vi "Prueba Trip Gap.vi"(11 "Class 2.lvclass":refnum<class "Class 2.lvclass">) -> (3 "Class 2.lvclass 2":refnum<class "Class 2.lvclass">)   [LabVIEW 2019, in "Class 2.lvclass"]
uses:
  Class 2.lvclass
  Class 2.lvclass/Class 2.ctl
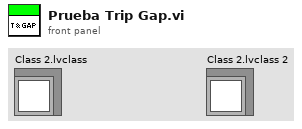
[diagram p1: front panel]
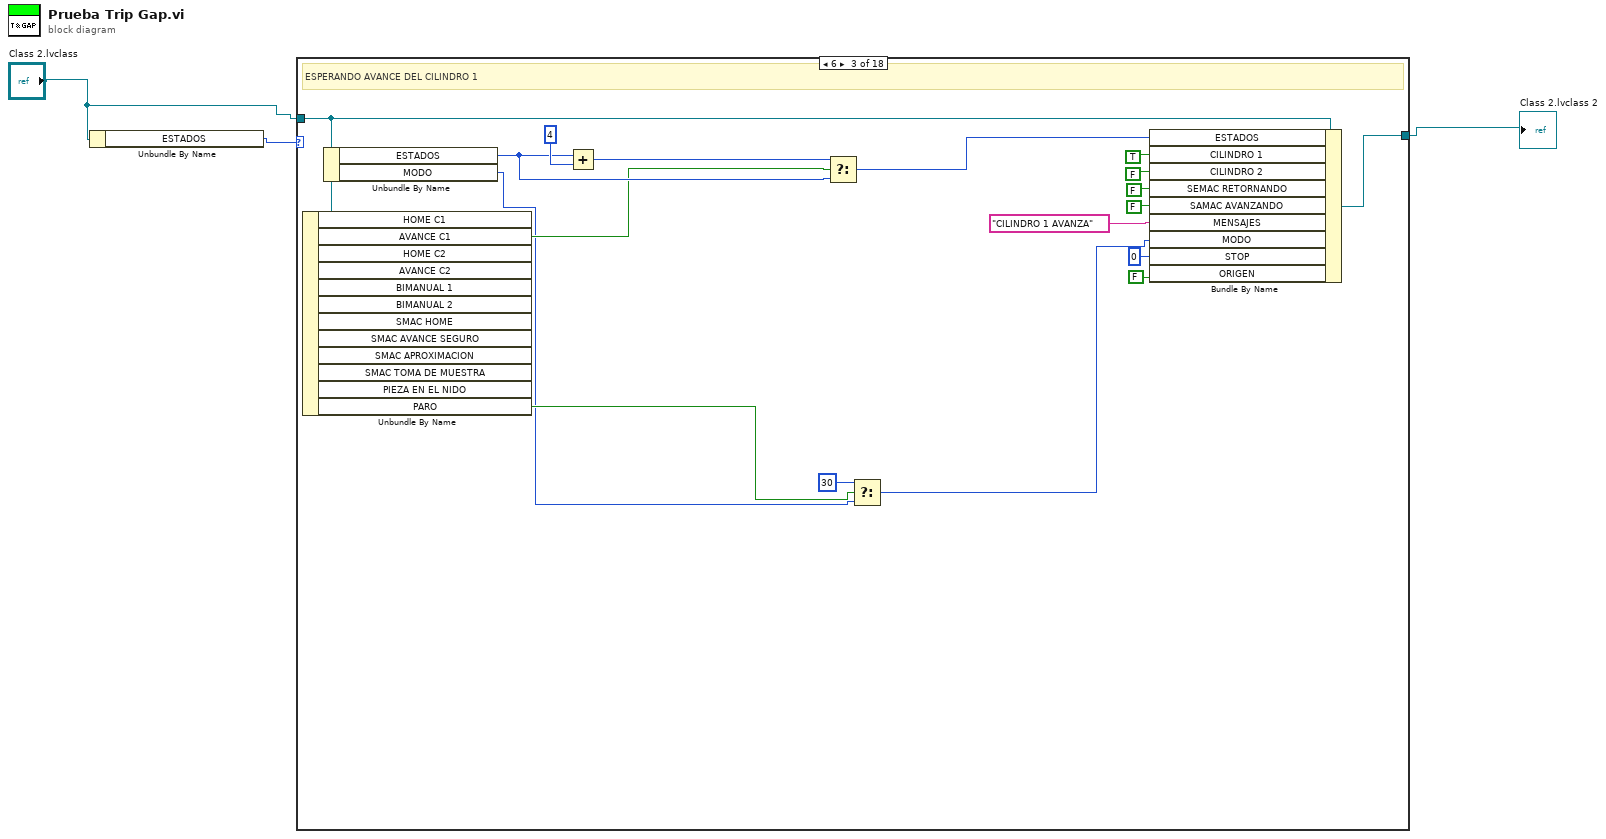
[diagram p0: block diagram]
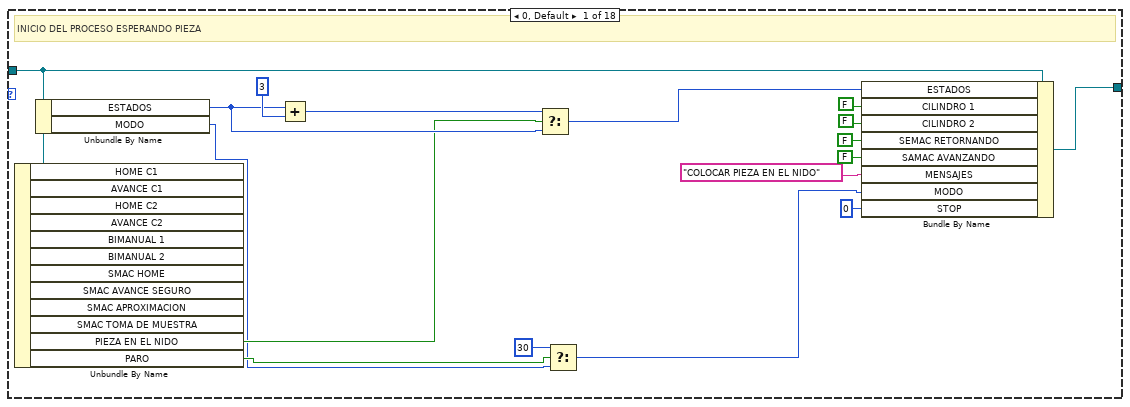
[diagram p2: hidden frame]
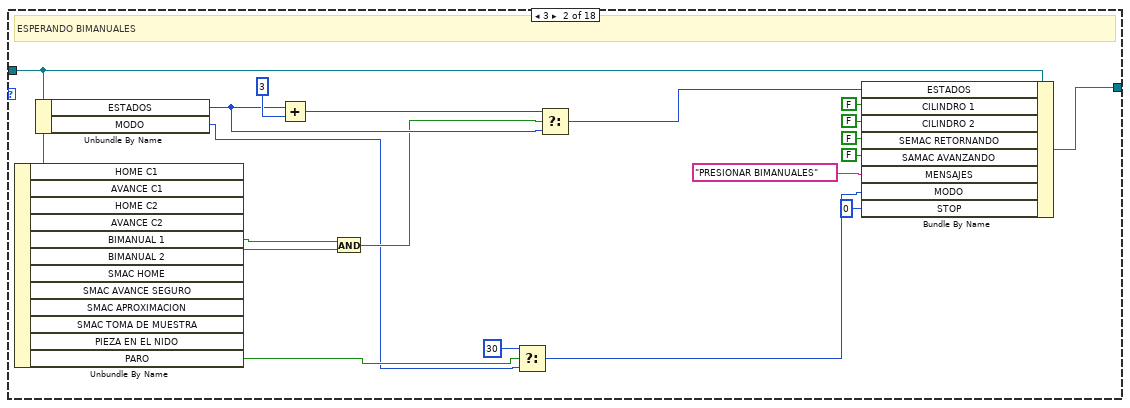
[diagram p3: hidden frame]
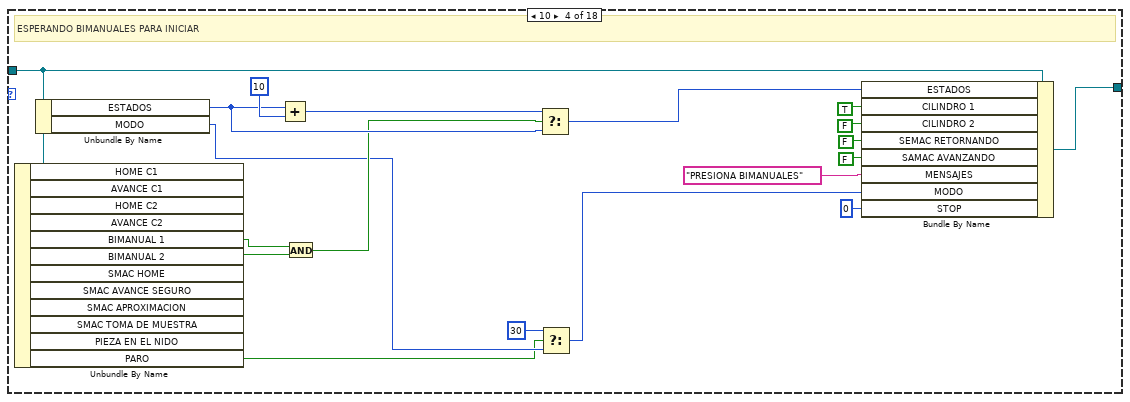
[diagram p4: hidden frame]
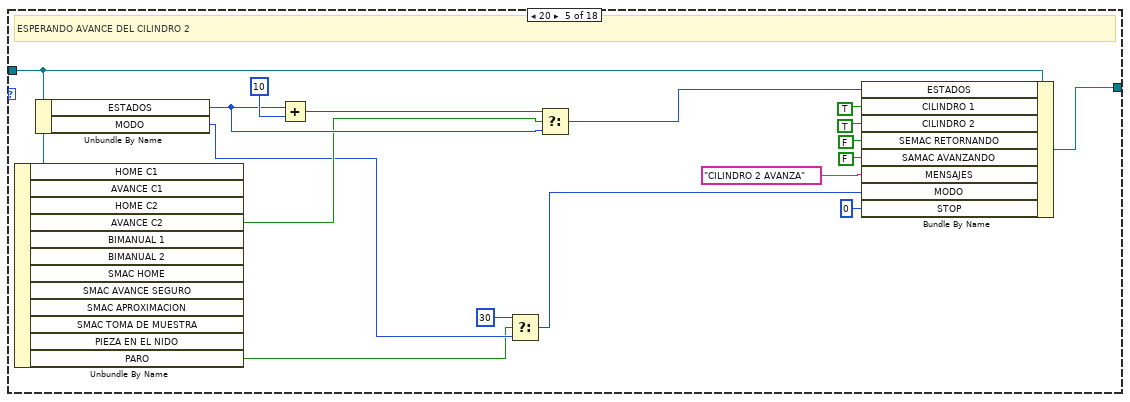
[diagram p5: hidden frame]
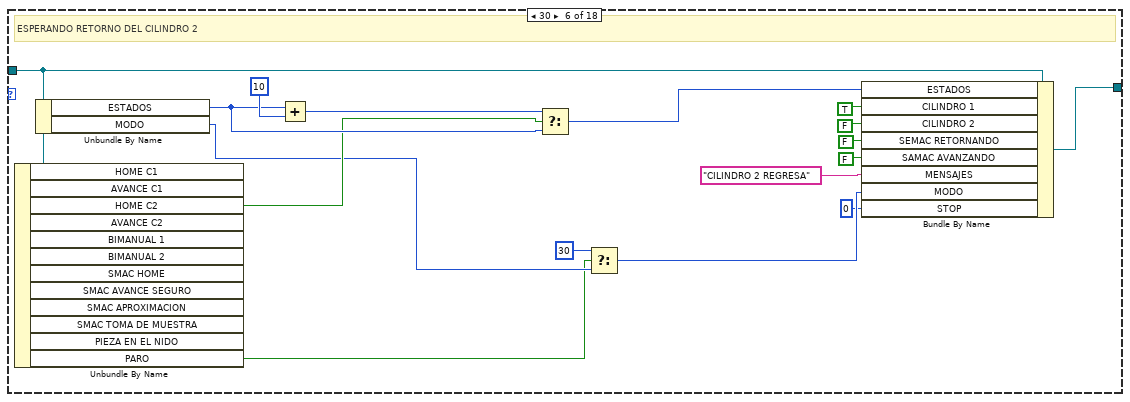
[diagram p6: hidden frame]
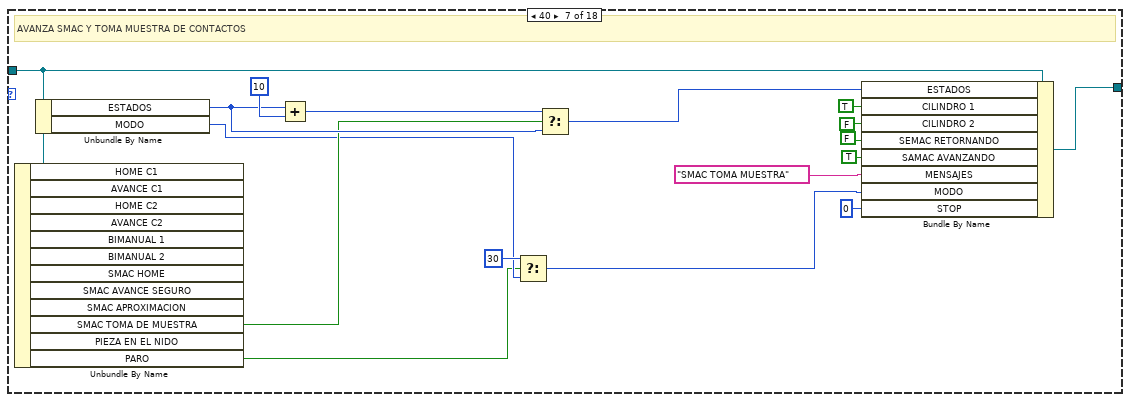
[diagram p7: hidden frame]
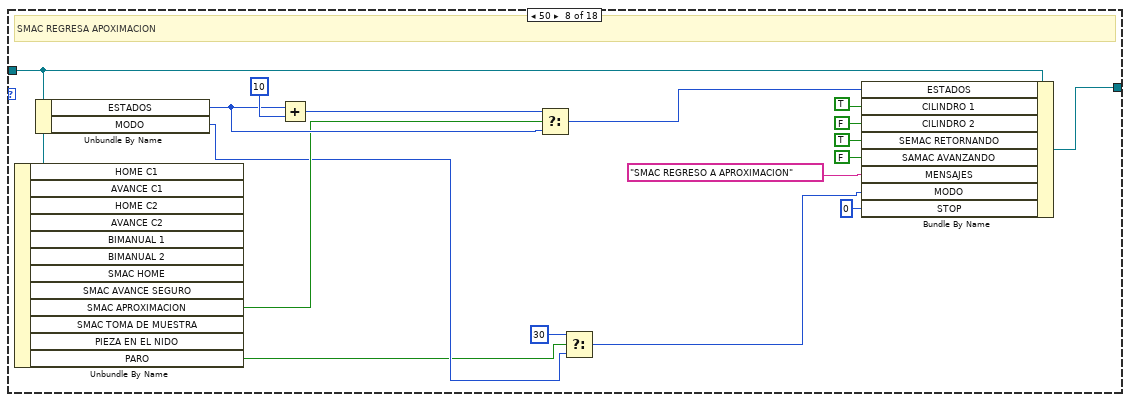
[diagram p8: hidden frame]
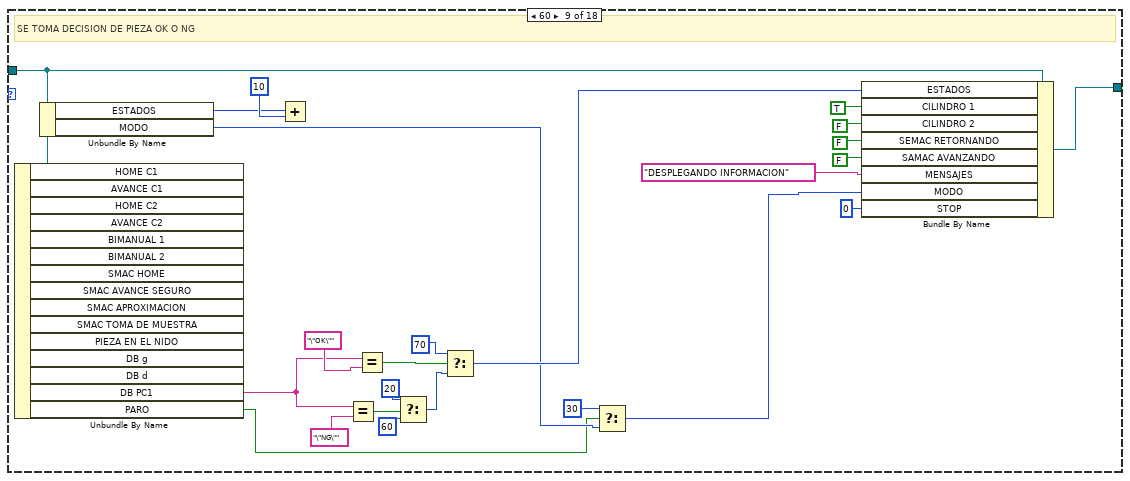
[diagram p9: hidden frame]
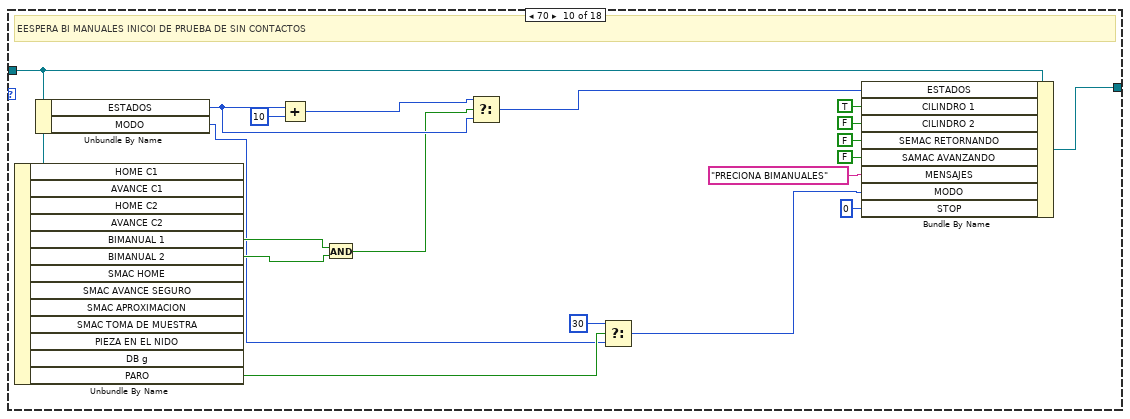
[diagram p10: hidden frame]
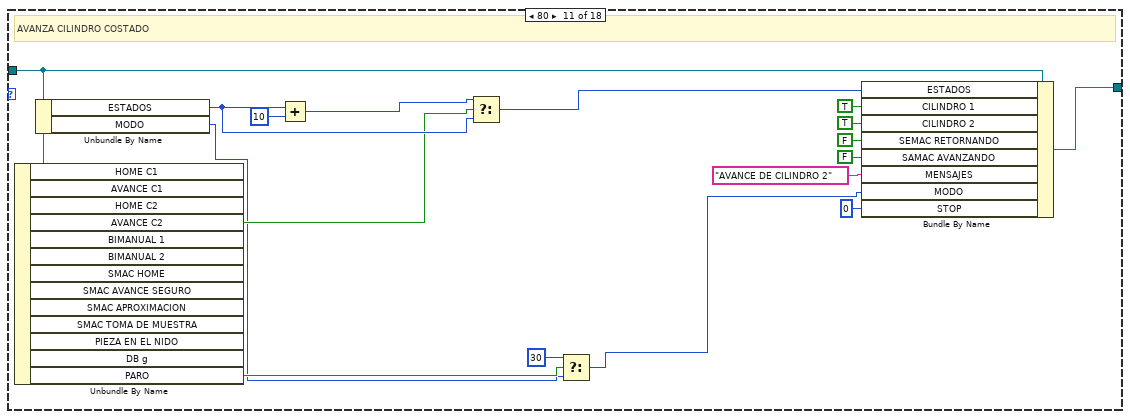
[diagram p11: hidden frame]
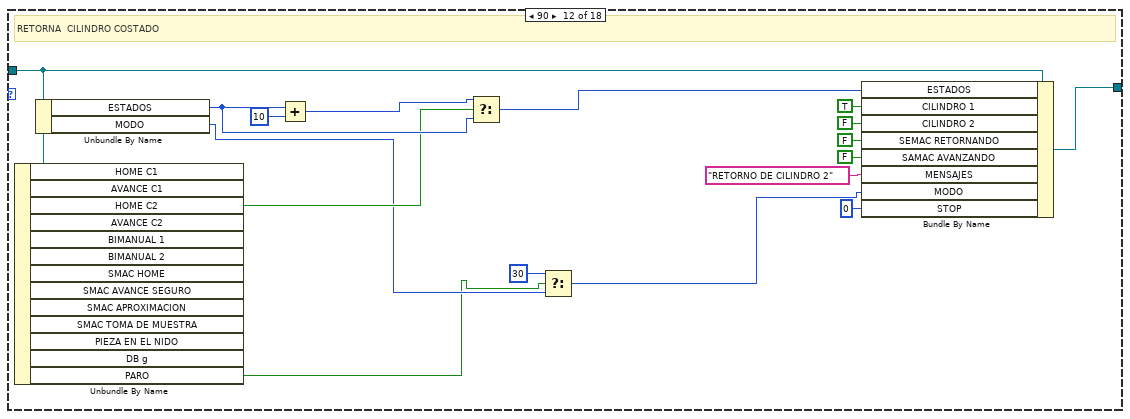
[diagram p12: hidden frame]
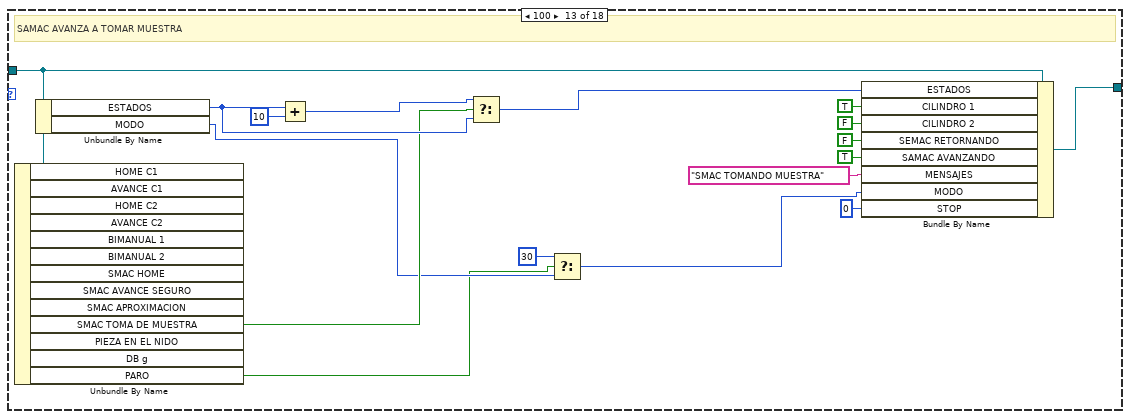
[diagram p13: hidden frame]
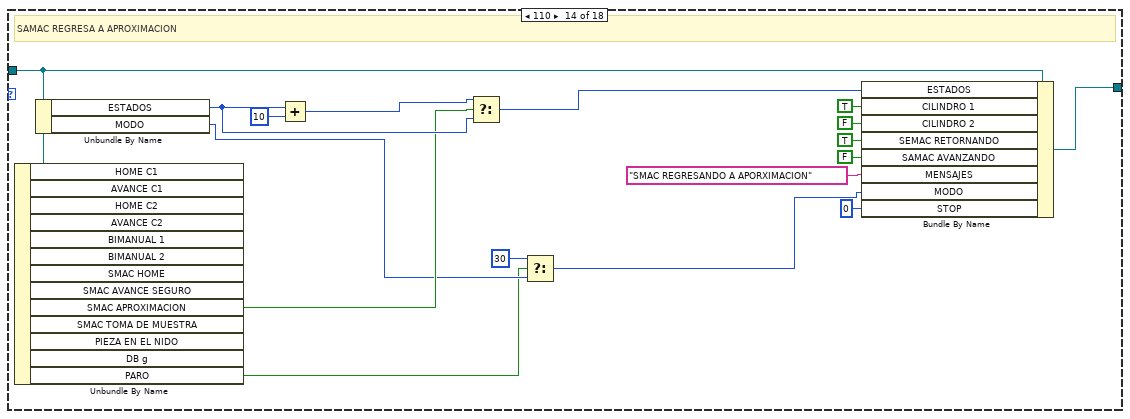
[diagram p14: hidden frame]
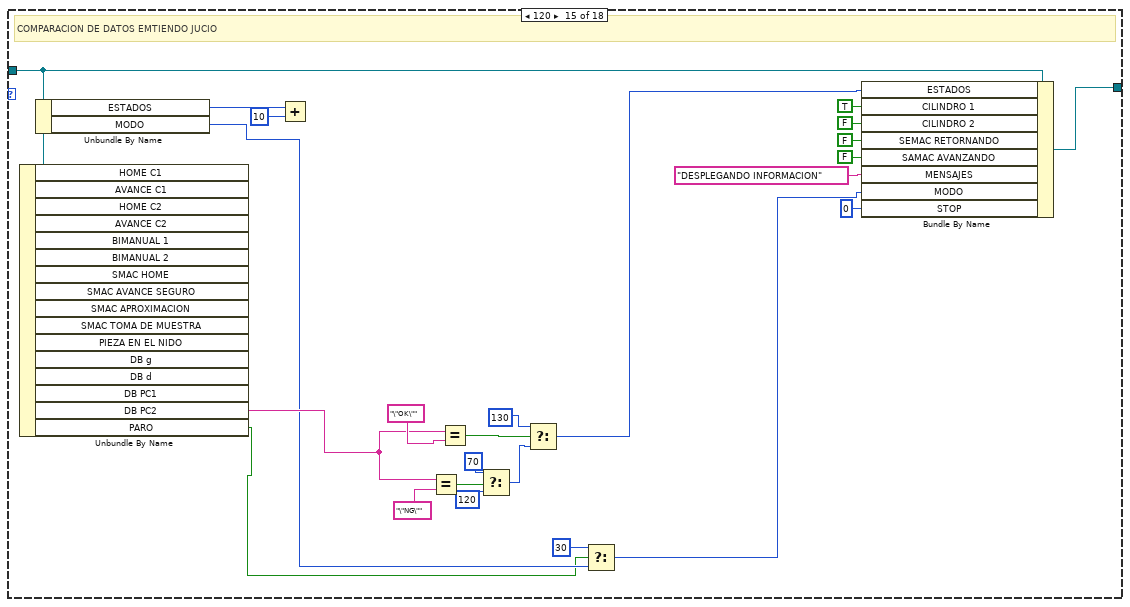
[diagram p15: hidden frame]
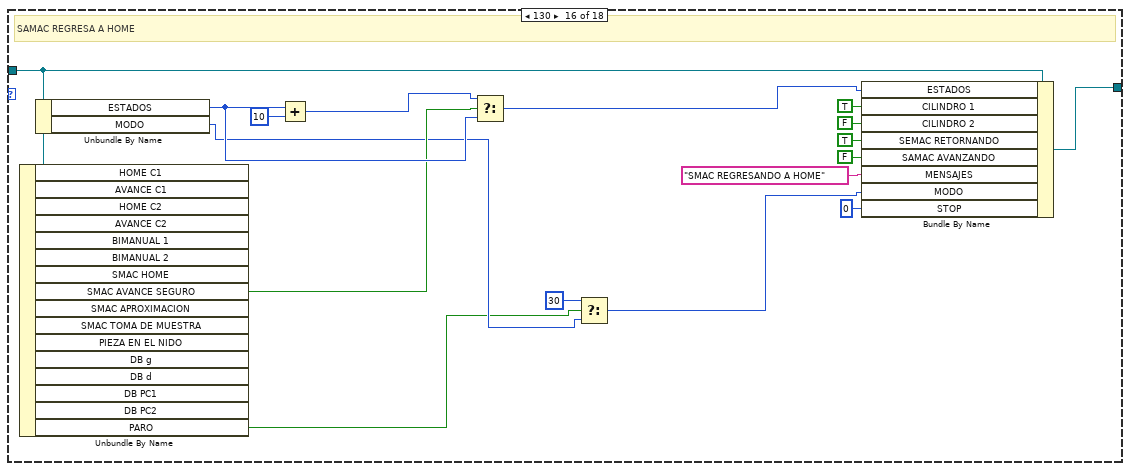
[diagram p16: hidden frame]
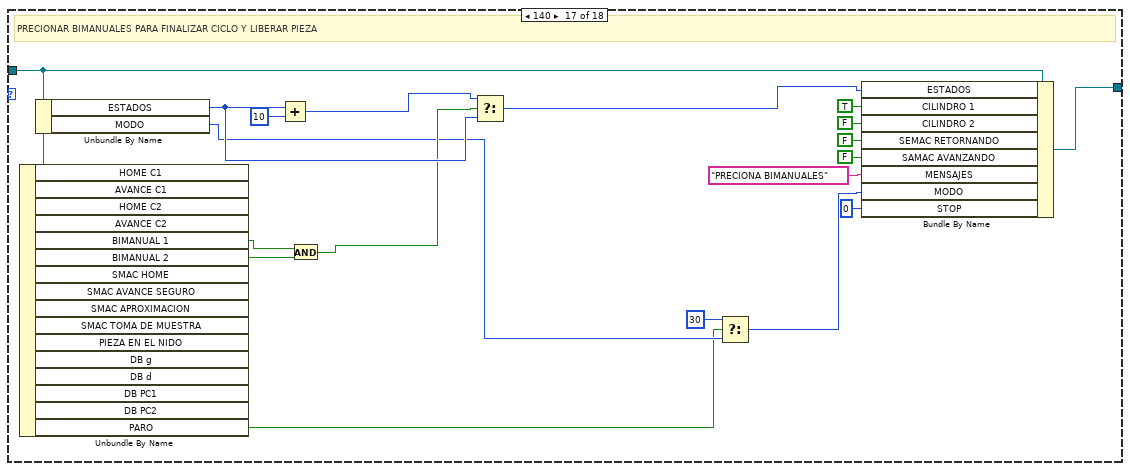
[diagram p17: hidden frame]
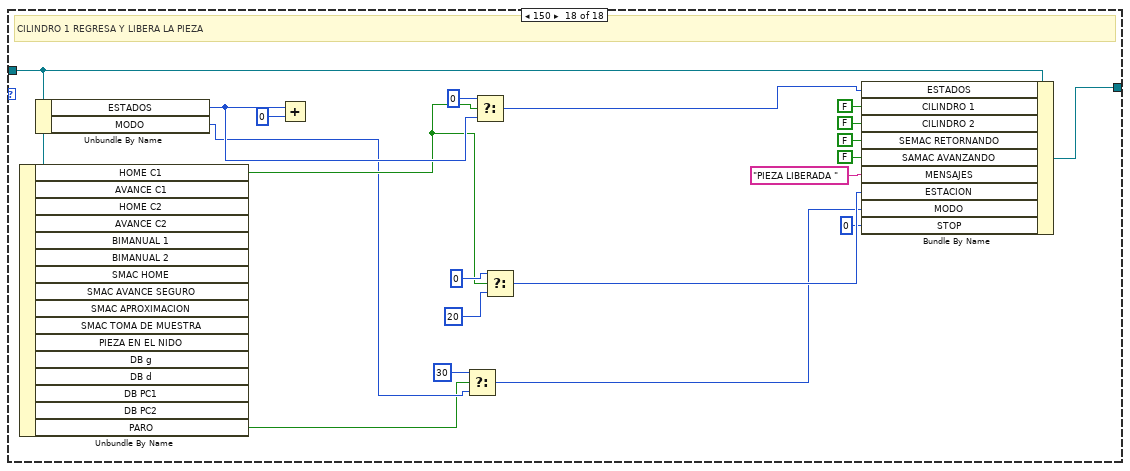
[diagram p18: hidden frame]
diagram:
  n1 = Unbundle By Name("Class 2.lvclass") -> ("ESTADOS"=w3:i16)
  n2 = case shown="6" w3 {
    tunnel: "Class 2.lvclass" -> [w15 w34 w52 w71 w88 w105 w122 w139 w166 w185 w202 w219 w236 w253 w277 w294 w313 w333]
    tunnel: [w20 w39 w57 w76 w93 w110 w127 w144 w168 w187 w204 w221 w238 w255 w279 w296 w315 w335] -> w1
    frame 0, Default {
      # "INICIO DEL PROCESO ESPERANDO PIEZA"
      n3 = Unbundle By Name(w15) -> ("PIEZA EN EL NIDO"=w13:bool, "PARO"=w5:bool)  [unwired: 10 out]
      n4 = Unbundle By Name(w15) -> ("ESTADOS"=w17:i16, "MODO"=w4:i16)
      n5 = Add(x=w17, y=i16 3) -> (x+y=w18:i16)
      n6 = Select(t=w18, s=w13, f=w17) -> (s? t:f=w16:i16)
      n7 = Select(t=i16 30, s=w5, f=w4) -> (s? t:f=w7:i16)
      n8 = Bundle By Name(cluster=w15, "ESTADOS"=w16, "CILINDRO 1"=FALSE ("SALIDAS.CILINDRO 1"), "CILINDRO 2"=FALSE ("SALIDAS.CILINDRO 2"), "SEMAC RETORNANDO"=FALSE ("SALIDAS.SEMAC RETORNANDO"), "SAMAC AVANZANDO"=FALSE ("SALIDAS.SAMAC AVANZANDO"), "MENSAJES"="COLOCAR PIEZA EN EL NIDO" ("SALIDAS.MENSAJES"), "MODO"=w7, "STOP"=i16 0 ("MAQ DE ESTADOS.STOP")) -> (w20:refnum<class "Class 2.lvclass">)
    }
    frame 3 {
      # "ESPERANDO BIMANUALES"
      n9 = Unbundle By Name(w34) -> ("BIMANUAL 1"=w28:bool, "BIMANUAL 2"=w27:bool, "PARO"=w22:bool)  [unwired: 9 out]
      n10 = Unbundle By Name(w34) -> ("ESTADOS"=w36:i16, "MODO"=w21:i16)
      n11 = Add(x=w36, y=i16 3) -> (x+y=w37:i16)
      n12 = And(x=w28, y=w27) -> (x .and. y?=w26:bool)
      n13 = Select(t=i16 30, s=w22, f=w21) -> (s? t:f=w24:i16)
      n14 = Select(t=w37, s=w26, f=w36) -> (s? t:f=w35:i16)
      n15 = Bundle By Name(cluster=w34, "ESTADOS"=w35, "CILINDRO 1"=FALSE ("SALIDAS.CILINDRO 1"), "CILINDRO 2"=FALSE ("SALIDAS.CILINDRO 2"), "SEMAC RETORNANDO"=FALSE ("SALIDAS.SEMAC RETORNANDO"), "SAMAC AVANZANDO"=FALSE ("SALIDAS.SAMAC AVANZANDO"), "MENSAJES"="PRESIONAR BIMANUALES" ("SALIDAS.MENSAJES"), "MODO"=w24, "STOP"=i16 0 ("MAQ DE ESTADOS.STOP")) -> (w39:refnum<class "Class 2.lvclass">)
    }
    frame 6 {
      # "ESPERANDO AVANCE DEL CILINDRO 1"
      n16 = Unbundle By Name(w52) -> ("AVANCE C1"=w46:bool, "PARO"=w42:bool)  [unwired: 10 out]
      n17 = Unbundle By Name(w52) -> ("ESTADOS"=w54:i16, "MODO"=w41:i16)
      n18 = Add(x=w54, y=i16 4) -> (x+y=w55:i16)
      n19 = Select(t=w55, s=w46, f=w54) -> (s? t:f=w53:i16)
      n20 = Select(t=i16 30, s=w42, f=w41) -> (s? t:f=w44:i16)
      n21 = Bundle By Name(cluster=w52, "ESTADOS"=w53, "CILINDRO 1"=TRUE ("SALIDAS.CILINDRO 1"), "CILINDRO 2"=FALSE ("SALIDAS.CILINDRO 2"), "SEMAC RETORNANDO"=FALSE ("SALIDAS.SEMAC RETORNANDO"), "SAMAC AVANZANDO"=FALSE ("SALIDAS.SAMAC AVANZANDO"), "MENSAJES"="CILINDRO 1 AVANZA" ("SALIDAS.MENSAJES"), "MODO"=w44, "STOP"=i16 0 ("MAQ DE ESTADOS.STOP"), "ORIGEN"=FALSE ("PROCESO.ORIGEN")) -> (w57:refnum<class "Class 2.lvclass">)
    }
    frame 10 {
      # "ESPERANDO BIMANUALES PARA INICIAR"
      n22 = Unbundle By Name(w71) -> ("BIMANUAL 1"=w65:bool, "BIMANUAL 2"=w64:bool, "PARO"=w58:bool)  [unwired: 9 out]
      n23 = Unbundle By Name(w71) -> ("ESTADOS"=w73:i16, "MODO"=w59:i16)
      n24 = Add(x=w73, y=i16 10) -> (x+y=w74:i16)
      n25 = And(x=w65, y=w64) -> (x .and. y?=w63:bool)
      n26 = Select(t=w74, s=w63, f=w73) -> (s? t:f=w72:i16)
      n27 = Select(t=i16 30, s=w58, f=w59) -> (s? t:f=w61:i16)
      n28 = Bundle By Name(cluster=w71, "ESTADOS"=w72, "CILINDRO 1"=TRUE ("SALIDAS.CILINDRO 1"), "CILINDRO 2"=FALSE ("SALIDAS.CILINDRO 2"), "SEMAC RETORNANDO"=FALSE ("SALIDAS.SEMAC RETORNANDO"), "SAMAC AVANZANDO"=FALSE ("SALIDAS.SAMAC AVANZANDO"), "MENSAJES"="PRESIONA BIMANUALES" ("SALIDAS.MENSAJES"), "MODO"=w61, "STOP"=i16 0 ("MAQ DE ESTADOS.STOP")) -> (w76:refnum<class "Class 2.lvclass">)
    }
    frame 20 {
      # "ESPERANDO AVANCE DEL CILINDRO 2"
      n29 = Unbundle By Name(w88) -> ("AVANCE C2"=w82:bool, "PARO"=w77:bool)  [unwired: 10 out]
      n30 = Unbundle By Name(w88) -> ("ESTADOS"=w90:i16, "MODO"=w78:i16)
      n31 = Add(x=w90, y=i16 10) -> (x+y=w91:i16)
      n32 = Select(t=i16 30, s=w77, f=w78) -> (s? t:f=w80:i16)
      n33 = Select(t=w91, s=w82, f=w90) -> (s? t:f=w89:i16)
      n34 = Bundle By Name(cluster=w88, "ESTADOS"=w89, "CILINDRO 1"=TRUE ("SALIDAS.CILINDRO 1"), "CILINDRO 2"=TRUE ("SALIDAS.CILINDRO 2"), "SEMAC RETORNANDO"=FALSE ("SALIDAS.SEMAC RETORNANDO"), "SAMAC AVANZANDO"=FALSE ("SALIDAS.SAMAC AVANZANDO"), "MENSAJES"="CILINDRO 2 AVANZA" ("SALIDAS.MENSAJES"), "MODO"=w80, "STOP"=i16 0 ("MAQ DE ESTADOS.STOP")) -> (w93:refnum<class "Class 2.lvclass">)
    }
    frame 30 {
      # "ESPERANDO RETORNO DEL CILINDRO 2"
      n35 = Unbundle By Name(w105) -> ("HOME C2"=w99:bool, "PARO"=w94:bool)  [unwired: 10 out]
      n36 = Unbundle By Name(w105) -> ("ESTADOS"=w107:i16, "MODO"=w95:i16)
      n37 = Add(x=w107, y=i16 10) -> (x+y=w108:i16)
      n38 = Select(t=w108, s=w99, f=w107) -> (s? t:f=w106:i16)
      n39 = Select(t=i16 30, s=w94, f=w95) -> (s? t:f=w97:i16)
      n40 = Bundle By Name(cluster=w105, "ESTADOS"=w106, "CILINDRO 1"=TRUE ("SALIDAS.CILINDRO 1"), "CILINDRO 2"=FALSE ("SALIDAS.CILINDRO 2"), "SEMAC RETORNANDO"=FALSE ("SALIDAS.SEMAC RETORNANDO"), "SAMAC AVANZANDO"=FALSE ("SALIDAS.SAMAC AVANZANDO"), "MENSAJES"="CILINDRO 2 REGRESA" ("SALIDAS.MENSAJES"), "MODO"=w97, "STOP"=i16 0 ("MAQ DE ESTADOS.STOP")) -> (w110:refnum<class "Class 2.lvclass">)
    }
    frame 40 {
      # "AVANZA SMAC Y TOMA MUESTRA DE CONTACTOS"
      n41 = Unbundle By Name(w122) -> ("SMAC TOMA DE MUESTRA"=w116:bool, "PARO"=w111:bool)  [unwired: 10 out]
      n42 = Unbundle By Name(w122) -> ("ESTADOS"=w124:i16, "MODO"=w112:i16)
      n43 = Add(x=w124, y=i16 10) -> (x+y=w125:i16)
      n44 = Select(t=i16 30, s=w111, f=w112) -> (s? t:f=w114:i16)
      n45 = Select(t=w125, s=w116, f=w124) -> (s? t:f=w123:i16)
      n46 = Bundle By Name(cluster=w122, "ESTADOS"=w123, "CILINDRO 1"=TRUE ("SALIDAS.CILINDRO 1"), "CILINDRO 2"=FALSE ("SALIDAS.CILINDRO 2"), "SEMAC RETORNANDO"=FALSE ("SALIDAS.SEMAC RETORNANDO"), "SAMAC AVANZANDO"=TRUE ("SALIDAS.SAMAC AVANZANDO"), "MENSAJES"="SMAC TOMA MUESTRA" ("SALIDAS.MENSAJES"), "MODO"=w114, "STOP"=i16 0 ("MAQ DE ESTADOS.STOP")) -> (w127:refnum<class "Class 2.lvclass">)
    }
    frame 50 {
      # "SMAC REGRESA APOXIMACION"
      n47 = Unbundle By Name(w139) -> ("SMAC APROXIMACION"=w133:bool, "PARO"=w128:bool)  [unwired: 10 out]
      n48 = Unbundle By Name(w139) -> ("ESTADOS"=w141:i16, "MODO"=w129:i16)
      n49 = Add(x=w141, y=i16 10) -> (x+y=w142:i16)
      n50 = Select(t=w142, s=w133, f=w141) -> (s? t:f=w140:i16)
      n51 = Select(t=i16 30, s=w128, f=w129) -> (s? t:f=w131:i16)
      n52 = Bundle By Name(cluster=w139, "ESTADOS"=w140, "CILINDRO 1"=TRUE ("SALIDAS.CILINDRO 1"), "CILINDRO 2"=FALSE ("SALIDAS.CILINDRO 2"), "SEMAC RETORNANDO"=TRUE ("SALIDAS.SEMAC RETORNANDO"), "SAMAC AVANZANDO"=FALSE ("SALIDAS.SAMAC AVANZANDO"), "MENSAJES"="SMAC REGRESO A APROXIMACION" ("SALIDAS.MENSAJES"), "MODO"=w131, "STOP"=i16 0 ("MAQ DE ESTADOS.STOP")) -> (w144:refnum<class "Class 2.lvclass">)
    }
    frame 60 {
      # "SE TOMA DECISION DE PIEZA OK O NG"
      n53 = Unbundle By Name(w166) -> ("DB PC1"=w150:string, "PARO"=w145:bool)  [unwired: 13 out]
      n54 = Unbundle By Name(w166) -> ("ESTADOS"=w159:i16, "MODO"=w146:i16)
      n55 = Add(x=w159, y=i16 10) -> ()  [unwired: 1 out]
      n56 = Equal?(x=w150, y="\"NG\"") -> (x = y?=w157:bool)
      n57 = Equal?(x=w150, y="\"OK\"") -> (x = y?=w158:bool)
      n58 = Select(t=i16 20 ("y"), s=w157, f=i16 60) -> (s? t:f=w154:i16)
      n59 = Select(t=i16 70, s=w158, f=w154) -> (s? t:f=w152:i16)
      n60 = Select(t=i16 30, s=w145, f=w146) -> (s? t:f=w148:i16)
      n61 = Bundle By Name(cluster=w166, "ESTADOS"=w152, "CILINDRO 1"=TRUE ("SALIDAS.CILINDRO 1"), "CILINDRO 2"=FALSE ("SALIDAS.CILINDRO 2"), "SEMAC RETORNANDO"=FALSE ("SALIDAS.SEMAC RETORNANDO"), "SAMAC AVANZANDO"=FALSE ("SALIDAS.SAMAC AVANZANDO"), "MENSAJES"="DESPLEGANDO INFORMACION" ("SALIDAS.MENSAJES"), "MODO"=w148, "STOP"=i16 0 ("MAQ DE ESTADOS.MODO")) -> (w168:refnum<class "Class 2.lvclass">)
    }
    frame 70 {
      # "EESPERA BI MANUALES INICOI DE PRUEBA DE SIN CONTACTOS"
      n62 = Unbundle By Name(w185) -> ("BIMANUAL 1"=w176:bool, "BIMANUAL 2"=w175:bool, "PARO"=w172:bool)  [unwired: 10 out]
      n63 = Unbundle By Name(w185) -> ("ESTADOS"=w178:i16, "MODO"=w171:i16)
      n64 = Add(x=w178, y=i16 10) -> (x+y=w177:i16)
      n65 = And(x=w176, y=w175) -> (x .and. y?=w174:bool)
      n66 = Select(t=w177, s=w174, f=w178) -> (s? t:f=w179:i16)
      n67 = Select(t=i16 30, s=w172, f=w171) -> (s? t:f=w170:i16)
      n68 = Bundle By Name(cluster=w185, "ESTADOS"=w179, "CILINDRO 1"=TRUE ("SALIDAS.CILINDRO 1"), "CILINDRO 2"=FALSE ("SALIDAS.CILINDRO 2"), "SEMAC RETORNANDO"=FALSE ("SALIDAS.SEMAC RETORNANDO"), "SAMAC AVANZANDO"=FALSE ("SALIDAS.SAMAC AVANZANDO"), "MENSAJES"="PRECIONA BIMANUALES" ("SALIDAS.MENSAJES"), "MODO"=w170, "STOP"=i16 0 ("MAQ DE ESTADOS.STOP")) -> (w187:refnum<class "Class 2.lvclass">)
    }
    frame 80 {
      # "AVANZA CILINDRO COSTADO"
      n69 = Unbundle By Name(w202) -> ("AVANCE C2"=w193:bool, "PARO"=w191:bool)  [unwired: 11 out]
      n70 = Unbundle By Name(w202) -> ("ESTADOS"=w195:i16, "MODO"=w190:i16)
      n71 = Add(x=w195, y=i16 10) -> (x+y=w194:i16)
      n72 = Select(t=w194, s=w193, f=w195) -> (s? t:f=w196:i16)
      n73 = Select(t=i16 30, s=w191, f=w190) -> (s? t:f=w189:i16)
      n74 = Bundle By Name(cluster=w202, "ESTADOS"=w196, "CILINDRO 1"=TRUE ("SALIDAS.CILINDRO 1"), "CILINDRO 2"=TRUE ("SALIDAS.CILINDRO 2"), "SEMAC RETORNANDO"=FALSE ("SALIDAS.SEMAC RETORNANDO"), "SAMAC AVANZANDO"=FALSE ("SALIDAS.SAMAC AVANZANDO"), "MENSAJES"="AVANCE DE CILINDRO 2" ("SALIDAS.MENSAJES"), "MODO"=w189, "STOP"=i16 0 ("MAQ DE ESTADOS.STOP")) -> (w204:refnum<class "Class 2.lvclass">)
    }
    frame 90 {
      # "RETORNA  CILINDRO COSTADO"
      n75 = Unbundle By Name(w219) -> ("HOME C2"=w210:bool, "PARO"=w206:bool)  [unwired: 11 out]
      n76 = Unbundle By Name(w219) -> ("ESTADOS"=w212:i16, "MODO"=w207:i16)
      n77 = Add(x=w212, y=i16 10) -> (x+y=w211:i16)
      n78 = Select(t=w211, s=w210, f=w212) -> (s? t:f=w213:i16)
      n79 = Select(t=i16 30, s=w206, f=w207) -> (s? t:f=w208:i16)
      n80 = Bundle By Name(cluster=w219, "ESTADOS"=w213, "CILINDRO 1"=TRUE ("SALIDAS.CILINDRO 1"), "CILINDRO 2"=FALSE ("SALIDAS.CILINDRO 2"), "SEMAC RETORNANDO"=FALSE ("SALIDAS.SEMAC RETORNANDO"), "SAMAC AVANZANDO"=FALSE ("SALIDAS.SAMAC AVANZANDO"), "MENSAJES"="RETORNO DE CILINDRO 2" ("SALIDAS.MENSAJES"), "MODO"=w208, "STOP"=i16 0 ("MAQ DE ESTADOS.STOP")) -> (w221:refnum<class "Class 2.lvclass">)
    }
    frame 100 {
      # "SAMAC AVANZA A TOMAR MUESTRA"
      n81 = Unbundle By Name(w236) -> ("SMAC TOMA DE MUESTRA"=w227:bool, "PARO"=w222:bool)  [unwired: 11 out]
      n82 = Unbundle By Name(w236) -> ("ESTADOS"=w229:i16, "MODO"=w223:i16)
      n83 = Add(x=w229, y=i16 10) -> (x+y=w228:i16)
      n84 = Select(t=w228, s=w227, f=w229) -> (s? t:f=w230:i16)
      n85 = Select(t=i16 30, s=w222, f=w223) -> (s? t:f=w225:i16)
      n86 = Bundle By Name(cluster=w236, "ESTADOS"=w230, "CILINDRO 1"=TRUE ("SALIDAS.CILINDRO 1"), "CILINDRO 2"=FALSE ("SALIDAS.CILINDRO 2"), "SEMAC RETORNANDO"=FALSE ("SALIDAS.SEMAC RETORNANDO"), "SAMAC AVANZANDO"=TRUE ("SALIDAS.SAMAC AVANZANDO"), "MENSAJES"="SMAC TOMANDO MUESTRA" ("SALIDAS.MENSAJES"), "MODO"=w225, "STOP"=i16 0 ("MAQ DE ESTADOS.STOP")) -> (w238:refnum<class "Class 2.lvclass">)
    }
    frame 110 {
      # "SAMAC REGRESA A APROXIMACION"
      n87 = Unbundle By Name(w253) -> ("SMAC APROXIMACION"=w244:bool, "PARO"=w239:bool)  [unwired: 11 out]
      n88 = Unbundle By Name(w253) -> ("ESTADOS"=w246:i16, "MODO"=w240:i16)
      n89 = Add(x=w246, y=i16 10) -> (x+y=w245:i16)
      n90 = Select(t=w245, s=w244, f=w246) -> (s? t:f=w247:i16)
      n91 = Select(t=i16 30, s=w239, f=w240) -> (s? t:f=w242:i16)
      n92 = Bundle By Name(cluster=w253, "ESTADOS"=w247, "CILINDRO 1"=TRUE ("SALIDAS.CILINDRO 1"), "CILINDRO 2"=FALSE ("SALIDAS.CILINDRO 2"), "SEMAC RETORNANDO"=TRUE ("SALIDAS.SEMAC RETORNANDO"), "SAMAC AVANZANDO"=FALSE ("SALIDAS.SAMAC AVANZANDO"), "MENSAJES"="SMAC REGRESANDO A APORXIMACION" ("SALIDAS.MENSAJES"), "MODO"=w242, "STOP"=i16 0 ("MAQ DE ESTADOS.STOP")) -> (w255:refnum<class "Class 2.lvclass">)
    }
    frame 120 {
      # "COMPARACION DE DATOS EMTIENDO JUCIO"
      n93 = Unbundle By Name(w277) -> ("DB PC2"=w262:string, "PARO"=w256:bool)  [unwired: 14 out]
      n94 = Unbundle By Name(w277) -> ("ESTADOS"=w271:i16, "MODO"=w257:i16)
      n95 = Add(x=w271, y=i16 10) -> ()  [unwired: 1 out]
      n96 = Equal?(x=w262, y="\"NG\"") -> (x = y?=w268:bool)
      n97 = Equal?(x=w262, y="\"OK\"") -> (x = y?=w269:bool)
      n98 = Select(t=i16 70 ("y"), s=w268, f=i16 120) -> (s? t:f=w265:i16)
      n99 = Select(t=i16 130, s=w269, f=w265) -> (s? t:f=w261:i16)
      n100 = Select(t=i16 30, s=w256, f=w257) -> (s? t:f=w259:i16)
      n101 = Bundle By Name(cluster=w277, "ESTADOS"=w261, "CILINDRO 1"=TRUE ("SALIDAS.CILINDRO 1"), "CILINDRO 2"=FALSE ("SALIDAS.CILINDRO 2"), "SEMAC RETORNANDO"=FALSE ("SALIDAS.SEMAC RETORNANDO"), "SAMAC AVANZANDO"=FALSE ("SALIDAS.SAMAC AVANZANDO"), "MENSAJES"="DESPLEGANDO INFORMACION" ("SALIDAS.MENSAJES"), "MODO"=w259, "STOP"=i16 0 ("MAQ DE ESTADOS.STOP")) -> (w279:refnum<class "Class 2.lvclass">)
    }
    frame 130 {
      # "SAMAC REGRESA A HOME"
      n102 = Unbundle By Name(w294) -> ("SMAC AVANCE SEGURO"=w285:bool, "PARO"=w280:bool)  [unwired: 14 out]
      n103 = Unbundle By Name(w294) -> ("ESTADOS"=w286:i16, "MODO"=w281:i16)
      n104 = Add(x=w286, y=i16 10) -> (x+y=w287:i16)
      n105 = Select(t=w287, s=w285, f=w286) -> (s? t:f=w288:i16)
      n106 = Select(t=i16 30, s=w280, f=w281) -> (s? t:f=w283:i16)
      n107 = Bundle By Name(cluster=w294, "ESTADOS"=w288, "CILINDRO 1"=TRUE ("SALIDAS.CILINDRO 1"), "CILINDRO 2"=FALSE ("SALIDAS.CILINDRO 2"), "SEMAC RETORNANDO"=TRUE ("SALIDAS.SEMAC RETORNANDO"), "SAMAC AVANZANDO"=FALSE ("SALIDAS.SAMAC AVANZANDO"), "MENSAJES"="SMAC REGRESANDO A HOME" ("SALIDAS.MENSAJES"), "MODO"=w283, "STOP"=i16 0 ("MAQ DE ESTADOS.STOP")) -> (w296:refnum<class "Class 2.lvclass">)
    }
    frame 140 {
      # "PRECIONAR BIMANUALES PARA FINALIZAR CICLO Y LIBERAR PIEZA"
      n108 = Unbundle By Name(w313) -> ("BIMANUAL 1"=w304:bool, "BIMANUAL 2"=w303:bool, "PARO"=w297:bool)  [unwired: 13 out]
      n109 = Unbundle By Name(w313) -> ("ESTADOS"=w305:i16, "MODO"=w298:i16)
      n110 = Add(x=w305, y=i16 10) -> (x+y=w306:i16)
      n111 = And(x=w304, y=w303) -> (x .and. y?=w302:bool)
      n112 = Select(t=w306, s=w302, f=w305) -> (s? t:f=w307:i16)
      n113 = Select(t=i16 30, s=w297, f=w298) -> (s? t:f=w300:i16)
      n114 = Bundle By Name(cluster=w313, "ESTADOS"=w307, "CILINDRO 1"=TRUE ("SALIDAS.CILINDRO 1"), "CILINDRO 2"=FALSE ("SALIDAS.CILINDRO 2"), "SEMAC RETORNANDO"=FALSE ("SALIDAS.SEMAC RETORNANDO"), "SAMAC AVANZANDO"=FALSE ("SALIDAS.SAMAC AVANZANDO"), "MENSAJES"="PRECIONA BIMANUALES" ("SALIDAS.MENSAJES"), "MODO"=w300, "STOP"=i16 0 ("MAQ DE ESTADOS.STOP")) -> (w315:refnum<class "Class 2.lvclass">)
    }
    frame 150 {
      # "CILINDRO 1 REGRESA Y LIBERA LA PIEZA"
      n115 = Unbundle By Name(w333) -> ("HOME C1"=w321:bool, "PARO"=w316:bool)  [unwired: 14 out]
      n116 = Unbundle By Name(w333) -> ("ESTADOS"=w326:i16, "MODO"=w317:i16)
      n117 = Add(x=w326, y=i16 0) -> ()  [unwired: 1 out]
      n118 = Select(t=i16 30, s=w316, f=w317) -> (s? t:f=w319:i16)
      n119 = Select(t=i16 0, s=w321, f=w326) -> (s? t:f=w327:i16)
      n120 = Select(t=i16 0, s=w321, f=i16 20 ("t")) -> (s? t:f=w322:i16)
      n121 = Bundle By Name(cluster=w333, "ESTADOS"=w327, "CILINDRO 1"=FALSE ("SALIDAS.CILINDRO 1"), "CILINDRO 2"=FALSE ("SALIDAS.CILINDRO 2"), "SEMAC RETORNANDO"=FALSE ("SALIDAS.SEMAC RETORNANDO"), "SAMAC AVANZANDO"=FALSE ("SALIDAS.SAMAC AVANZANDO"), "MENSAJES"="PIEZA LIBERADA " ("SALIDAS.MENSAJES"), "ESTACION"=w322, "MODO"=w319, "STOP"=i16 0 ("MAQ DE ESTADOS.STOP")) -> (w335:refnum<class "Class 2.lvclass">)
    }
  }
  "Class 2.lvclass 2" <- w1
